vi "Restart.vi"(5 "Timeout msec (180000)":u32=180000 caption="Timeout (180000 ms)", 6 "Wait until complete (true)":bool=TRUE, 7 "error in (no error)":errorcluster, 8 "Flush DNS (false)":bool, 9 "Install mode (false)":bool, 10 "RT Management in":refnum<class "RT Management.lvclass">) -> (0 "error out":errorcluster, 3 "RT Management out":refnum<class "RT Management.lvclass">)   [LabVIEW 2015, in "RT Management.lvlib" / "RT Management.lvclass"]
doc: "Reboots the RT target."
uses:
  RT Management.lvclass
  RT Management.lvclass/RT Management.ctl
  Get SysCfg Session.vi
  Get Restart needed.vi
  Set SysCfg Session.vi
  Set Address.vi
  Set Restart needed.vi
  <vilib>/nisyscfg/nisyscfg.lvlib
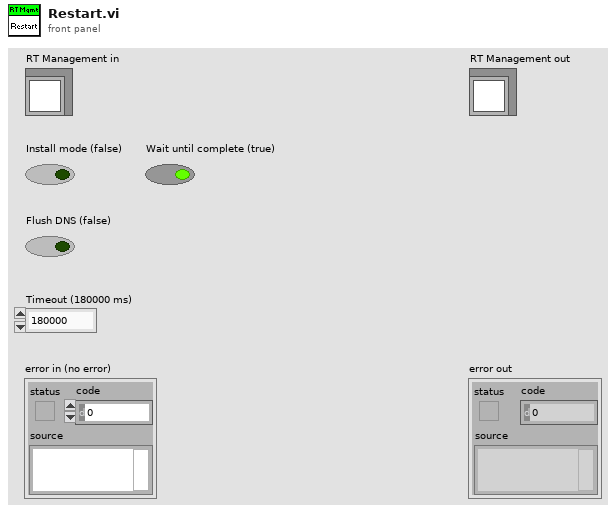
[diagram p1: front panel]
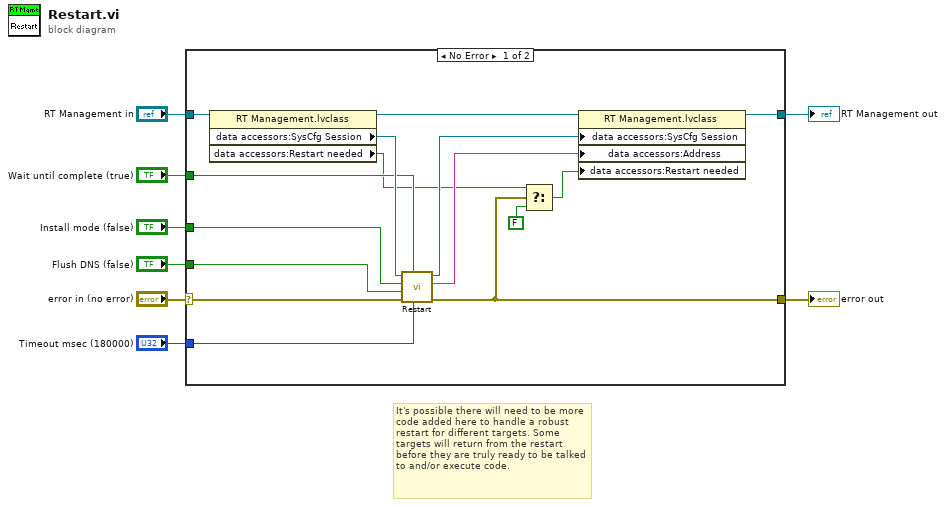
[diagram p0: block diagram]
diagram:
  # "It's possible there will need to be more code added here to handle a robust restart for different targets. Some targets will return from the restart before they are truly ready to be talked to and/or execute code."
  n1 = case shown="No Error" "error in (no error)" {
    selector: "error in (no error)" -> [w22 w25]
    tunnel: [w12 w25] -> w7
    tunnel: [w13 w24] -> w5
    tunnel: "RT Management in" -> [w23 w24]
    tunnel: "Timeout msec (180000)" -> [w14 _]
    tunnel: "Wait until complete (true)" -> [w18 _]
    tunnel: "Install mode (false)" -> [w17 _]
    tunnel: "Flush DNS (false)" -> [w16 _]
    frame No Error {
      n2 = property class="RT Management.lvclass"(reference=w23) -> (reference out=w19:refnum<class "RT Management.lvclass">, "data accessors:SysCfg Session"=w21:refnum<k21>, "data accessors:Restart needed"=w11:bool)  [unwired: 1 in, 1 out]
      n3 = call <vilib>:"Restart.vi"("Timeout (180,000 ms)"=w14, "Wait Until Complete (T)"=w18, "error in (no error)"=w22, "Flush DNS (F)"=w16, "Install Mode (F)"=w17, "Session in"=w21) -> ("error out"=w12:errorcluster, "New IP Address"=w15:string, "Session out"=w20:refnum<k21>)  [unwired: 3 in]
      n4 = Select(t=w11, s=w12, f=FALSE ("Restart needed")) -> (s? t:f=w10:bool)
      n5 = property class="RT Management.lvclass"(reference=w19, "data accessors:SysCfg Session"=w20, "data accessors:Address"=w15, "data accessors:Restart needed"=w10) -> (reference out=w13:refnum<class "RT Management.lvclass">)  [unwired: 1 in, 1 out]
    }
    frame Error {
    }
  }
  "error out" <- w7
  "RT Management out" <- w5
